vi "PGBackground.vi"(8 "error in":errorcluster, 11 "VISA resource name":refnum<visa-resource-name>) -> (0 "error out":errorcluster, 3 "VISA resource name out":refnum<visa-resource-name>)   [LabVIEW 2018]
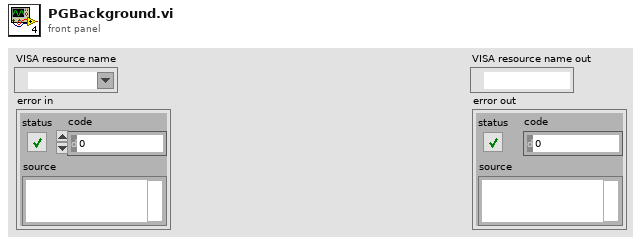
[diagram p1: front panel]
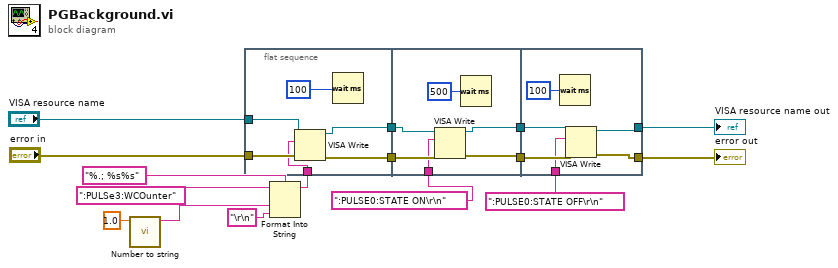
[diagram p0: block diagram]
diagram:
  n1 = call "Number to string.vi"("Numeric"=1.0) -> ("Shortest String"=w12:string)  [unwired: 10 in]
  n2 = flat-sequence {
    tunnel: "VISA resource name" -> [w22]
    tunnel: "error in" -> [w21]
    tunnel: w9 -> [w20]
    tunnel: [w19] -> w6
    tunnel: [w18] -> w5
    tunnel: w6 -> [w28]
    tunnel: w5 -> [w26]
    tunnel: ":PULSE0:STATE ON\r\n" ("format string") -> [w24]
    tunnel: [w27] -> w3
    tunnel: [w25] -> w2
    tunnel: [w31] -> w7
    tunnel: [w32] -> w8
    tunnel: w3 -> [w33]
    tunnel: w2 -> [w34]
    tunnel: ":PULSE0:STATE OFF\r\n" ("format string") -> [w30]
    frame #0 {
      n3 = VISA Write(VISA resource name=w22, write buffer=w20, error in (no error)=w21) -> (VISA resource name out=w19:refnum<visa-resource-name>, error out=w18:errorcluster)  [unwired: 1 out]
      n4 = Wait (ms)(milliseconds to wait=u32 100) -> ()  [unwired: 1 out]
    }
    frame #1 {
      n5 = VISA Write(VISA resource name=w28, write buffer=w24, error in (no error)=w26) -> (VISA resource name out=w27:refnum<visa-resource-name>, error out=w25:errorcluster)  [unwired: 1 out]
      n6 = Wait (ms)(milliseconds to wait=u32 500) -> ()  [unwired: 1 out]
    }
    frame #2 {
      n7 = Wait (ms)(milliseconds to wait=u32 100) -> ()  [unwired: 1 out]
      n8 = VISA Write(VISA resource name=w33, write buffer=w30, error in (no error)=w34) -> (VISA resource name out=w32:refnum<visa-resource-name>, error out=w31:errorcluster)  [unwired: 1 out]
    }
  }
  n9 = Format Into String(format string="%.; %s%s", initial string=":PULSe3:WCOunter" ("format string"), w12, "\r\n" ("format string")) -> (resulting string=w9:string)  [unwired: 1 in, 1 out]
  "VISA resource name out" <- w8
  "error out" <- w7
